vi "Phase XY Stats.vi"(8 "Feedback In":T1, 9 "Heel Strike?":bool, 10 "Y":dbl, 11 "X":dbl) -> (0 "Feedback Out":T1)   [LabVIEW 2018]
uses:
  Phase Calculator Feedback Cluster.ctl
  <vilib>/ptbypt/NI_PtbyPt.lvlib
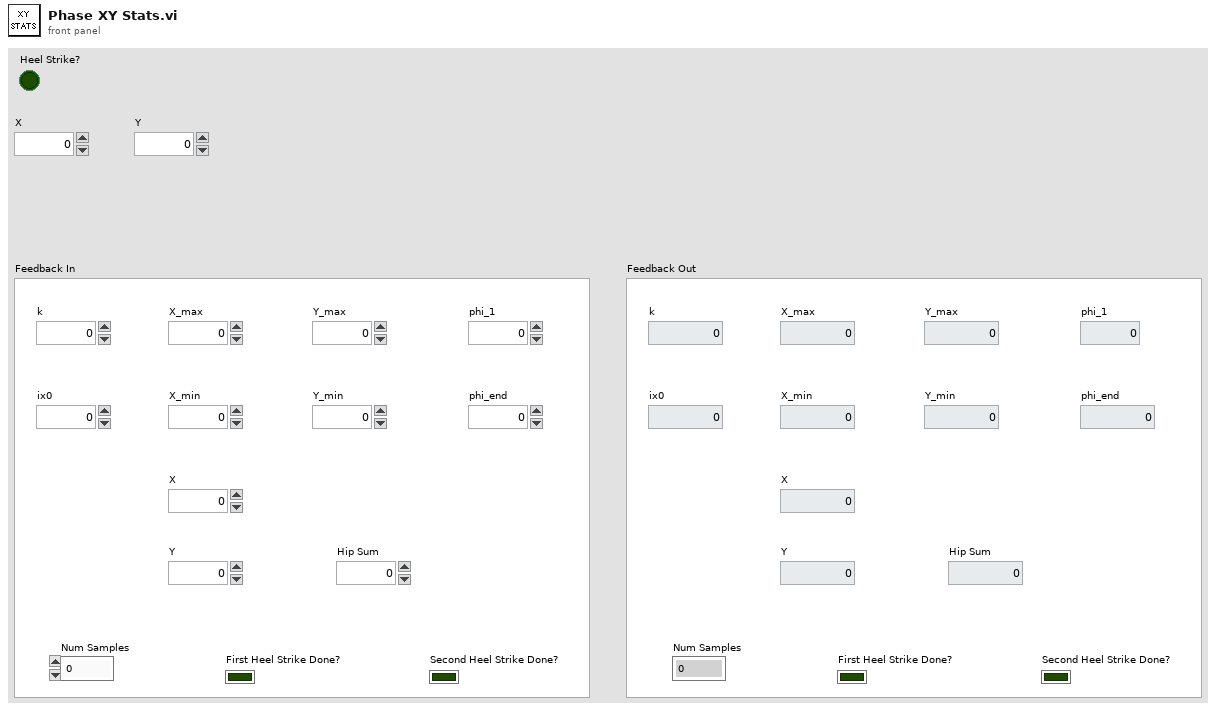
[diagram p1: front panel]
types:
  T1 = typedef "Phase Calculator Feedback Cluster.ctl" = cluster{"k":dbl, "ix0":dbl, "X_max":dbl, "X_min":dbl, "Y_max":dbl, "Y_min":dbl, "Y":dbl, "Hip Sum":dbl, "Num Samples":dbl, "First Heel Strike Done?":bool, "Second Heel Strike Done?":bool, "phi_1":dbl, "phi_end":dbl, "X":dbl}
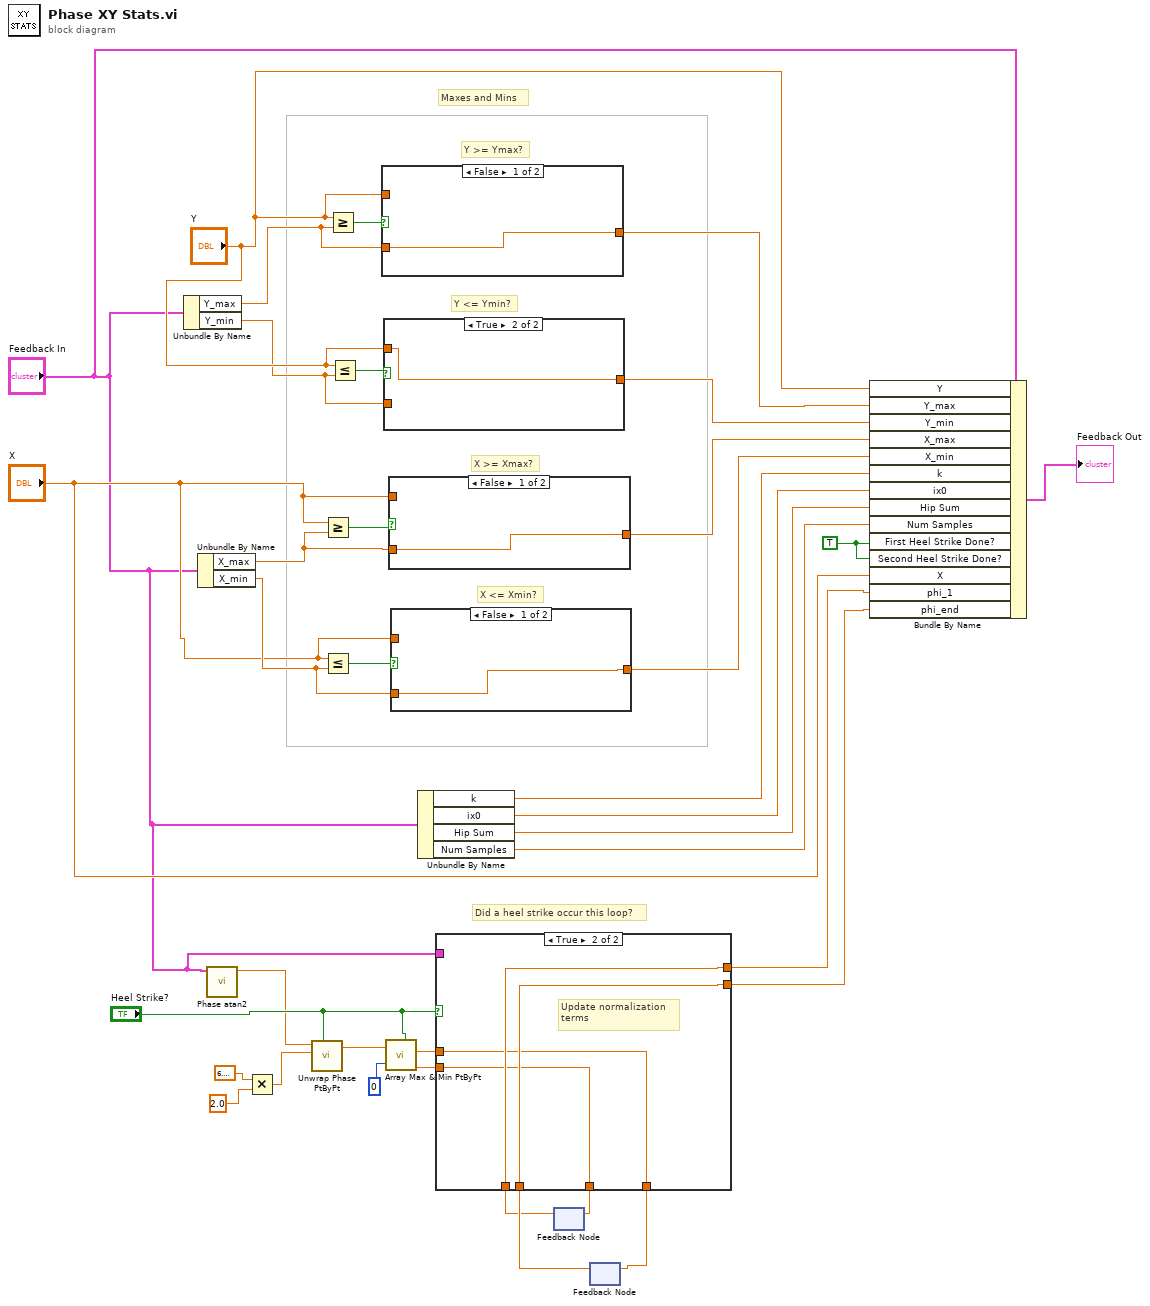
[diagram p0: block diagram]
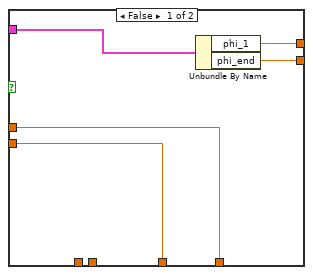
[diagram p2: hidden frame]
diagram:
  w18 = TRUE ("First Heel Strike Done?")
  # "Did a heel strike occur this loop?"
  # "Y <= Ymin?"
  # "Y >= Ymax?"
  # "X <= Xmin?"
  # "X >= Xmax?"
  # "Maxes and Mins"
  n1 = Unbundle By Name("Feedback In") -> ("Y_max"=w29:dbl, "Y_min"=w27:dbl)
  n2 = Unbundle By Name("Feedback In") -> ("X_max"=w34:dbl, "X_min"=w32:dbl)
  n3 = call "Phase atan2.vi"("Feedback In"="Feedback In") -> ("atan2(y,x)"=w4:dbl)  [unwired: 10 in]
  n4 = Multiply(x=6.283185307179586, y=2.0) -> (x*y=w2:dbl)
  n5 = call <vilib>:"Unwrap Phase PtByPt.vi"("initialize"="Heel Strike?", "wrap base"=w2, "phase"=w4) -> ("unwrapped phase"=w6:dbl)  [unwired: 8 in]
  n6 = Greater Or Equal?(x="X", y=w34) -> (x >= y?=w35:bool)
  n7 = Less Or Equal?(x="X", y=w32) -> (x <= y?=w33:bool)
  n8 = Greater Or Equal?(x="Y", y=w29) -> (x >= y?=w30:bool)
  n9 = Less Or Equal?(x="Y", y=w27) -> (x <= y?=w31:bool)
  n10 = case shown="False" w30 {
    tunnel: "Y" -> [_ w38]
    tunnel: w29 -> [w37 _]
    tunnel: [w37 w38] -> w26
    frame False {
    }
    frame True {
    }
  }
  n11 = case shown="True" w31 {
    tunnel: "Y" -> [_ w40]
    tunnel: w27 -> [w39 _]
    tunnel: [w39 w40] -> w25
    frame False {
    }
    frame True {
    }
  }
  n12 = call <vilib>:"Array Max & Min PtByPt.vi"("input data point"=w6, "sample length"=0, "initialize"="Heel Strike?") -> ("max value"=w12:dbl, "min value"=w11:dbl)  [unwired: 3 out]
  n13 = case shown="False" w35 {
    tunnel: "X" -> [_ w42]
    tunnel: w34 -> [w41 _]
    tunnel: [w41 w42] -> w24
    frame False {
    }
    frame True {
    }
  }
  n14 = case shown="False" w33 {
    tunnel: "X" -> [_ w44]
    tunnel: w32 -> [w43 _]
    tunnel: [w43 w44] -> w23
    frame False {
    }
    frame True {
    }
  }
  n15 = Unbundle By Name("Feedback In") -> ("k"=w22:dbl, "ix0"=w21:dbl, "Hip Sum"=w20:dbl, "Num Samples"=w19:dbl)
  n16 = feedback #1() -> (w7:dbl)  [unwired: 1 in]
  n17 = feedback #2() -> (w8:dbl)  [unwired: 1 in]
  n18 = case shown="True" "Heel Strike?" {
    tunnel: [w49 w52] -> w14
    tunnel: "Feedback In" -> [w48 _]
    tunnel: [w47 w53] -> w13
    tunnel: w12 -> [w45 w51]
    tunnel: w11 -> [w46 w50]
    tunnel: [w46 w50] -> w10
    tunnel: [w45 w51] -> w9
    tunnel: w8 -> [_ w53]
    tunnel: w7 -> [_ w52]
    frame False {
      n19 = Unbundle By Name(w48) -> ("phi_1"=w49:dbl, "phi_end"=w47:dbl)
    }
    frame True {
      # "Update normalization \nterms"
    }
  }
  n20 = feedback-in #1(w10) -> ()
  n21 = feedback-in #2(w9) -> ()
  n22 = Bundle By Name(cluster="Feedback In", "Y"="Y", "Y_max"=w26, "Y_min"=w25, "X_max"=w24, "X_min"=w23, "k"=w22, "ix0"=w21, "Hip Sum"=w20, "Num Samples"=w19, "First Heel Strike Done?"=w18, "Second Heel Strike Done?"=w18, "X"="X", "phi_1"=w14, "phi_end"=w13) -> (→"Feedback Out":T1)
